vi "Statistics.vi"() -> ()   [LabVIEW 2022 SP3]
uses:
  <vilib>/gmath/NI_Gmath.lvlib
panel:
  out "Number of Combinations":dbl
  in  "?":u16(ring) items=["Order Matters", "Order Doesn't Matter"]
  in  "?":u16(ring) items=["Samples Can Repeat", "Samples Cannot Repeat"]
  in  "Total Objects":dbl
  in  "Selected Objects":dbl
  # "Number of Combinations:\nFor a set of objects you wish to select from,\nthe following will calculate the number of unique\ncombinations. Set the conditions, total number of\nobjects, and number of selected objects."
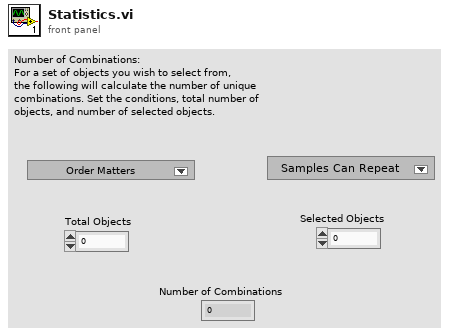
[diagram p1: front panel]
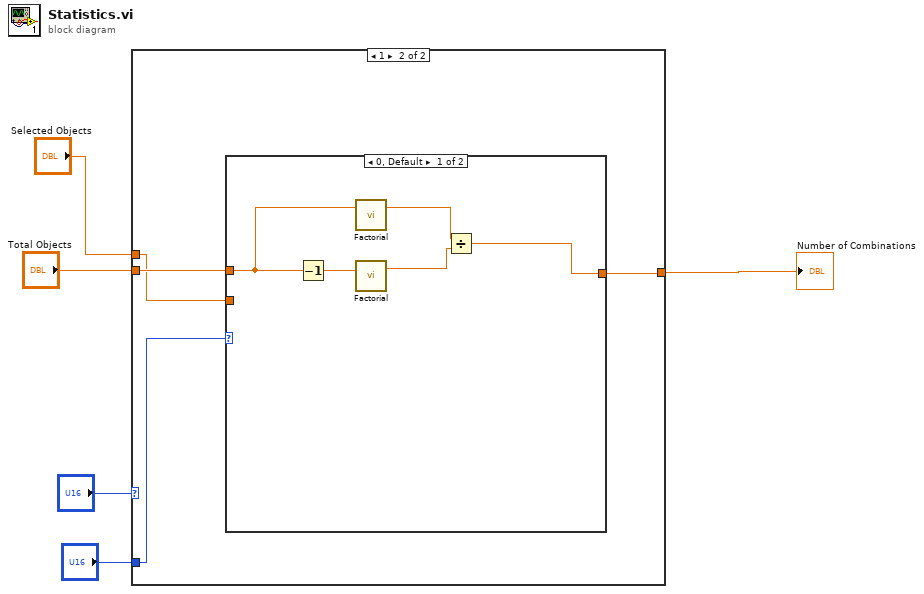
[diagram p0: block diagram]
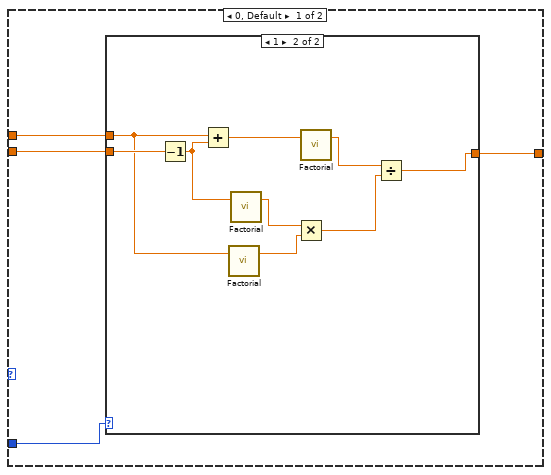
[diagram p2: hidden frame]
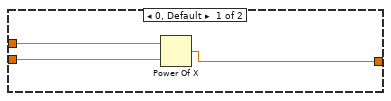
[diagram p3: hidden frame]
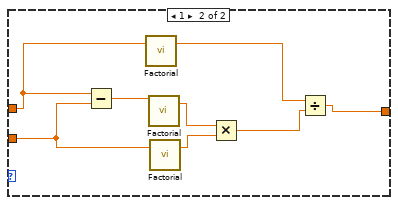
[diagram p4: hidden frame]
diagram:
  n1 = case shown="1" "?" {
    tunnel: "?" -> [w9 w25]
    tunnel: "Total Objects" -> [w8 w24]
    tunnel: "Selected Objects" -> [w7 w22]
    tunnel: [w6 w23] -> w1
    frame 0, Default {
      n2 = case shown="1" w9 {
        tunnel: w8 -> [w12 w21]
        tunnel: w7 -> [w11 w16]
        tunnel: [w10 w13] -> w6
        frame 0, Default {
          n3 = Power Of X(1:w12, 2:w11) -> (0:w10:dbl)
        }
        frame 1 {
          n4 = Decrement(x=w21) -> (x-1=w19:dbl)
          n5 = Add(x=w16, y=w19) -> (x+y=w20:dbl)
          n6 = call <vilib>:"Factorial.vi"("n"=w16) -> ("n!"=w17:dbl)  [unwired: 2 in]
          n7 = call <vilib>:"Factorial.vi"("n"=w19) -> ("n!"=w18:dbl)  [unwired: 2 in]
          n8 = Multiply(x=w18, y=w17) -> (x*y=w14:dbl)
          n9 = call <vilib>:"Factorial.vi"("n"=w20) -> ("n!"=w15:dbl)  [unwired: 2 in]
          n10 = Divide(x=w15, y=w14) -> (x/y=w13:dbl)
        }
      }
    }
    frame 1 {
      n11 = case shown="0, Default" w25 {
        tunnel: w24 -> [w29 w38]
        tunnel: [w26 w33] -> w23
        tunnel: w22 -> [_ w37]
        frame 0, Default {
          n12 = Decrement(x=w29) -> (x-1=w30:dbl)
          n13 = call <vilib>:"Factorial.vi"("n"=w29) -> ("n!"=w28:dbl)  [unwired: 2 in]
          n14 = call <vilib>:"Factorial.vi"("n"=w30) -> ("n!"=w27:dbl)  [unwired: 2 in]
          n15 = Divide(x=w28, y=w27) -> (x/y=w26:dbl)
        }
        frame 1 {
          n16 = Subtract(x=w38, y=w37) -> (x-y=w36:dbl)
          n17 = call <vilib>:"Factorial.vi"("n"=w38) -> ("n!"=w32:dbl)  [unwired: 2 in]
          n18 = call <vilib>:"Factorial.vi"("n"=w36) -> ("n!"=w35:dbl)  [unwired: 2 in]
          n19 = call <vilib>:"Factorial.vi"("n"=w37) -> ("n!"=w34:dbl)  [unwired: 2 in]
          n20 = Multiply(x=w35, y=w34) -> (x*y=w31:dbl)
          n21 = Divide(x=w32, y=w31) -> (x/y=w33:dbl)
        }
      }
    }
  }
  "Number of Combinations" <- w1
